vi "ULx Write (Digital Wfm 1Chan 1Samp).vi"(0 "task in":refnum<k24>, 1 "auto start":bool=TRUE, 7 "data":digitalwaveform(waveform)={"t0"=timestamp(0 s since 1904-01-01), "dt"=0.0, "Y"={"transitions"=[], "data"=[]}, "error"={"status"=FALSE, "code"=37421928, "source"=""}}, 9 "timeout":dbl=10.0 format="%_4g", 11 "error in":errorcluster) -> (4 "task out":refnum<k24>, 10 "number of samples written per channel":u32, 15 "error out":errorcluster)   [LabVIEW 2020]
doc: "Writes a digital waveform that contains a single sample to a task that contains a single digital output channel."
uses:
  C:/Users/William/Documents/LV 2020 builds/LeaktestDAQ/Source-v33/ULx_LV.dll
  ULx_LV.dll
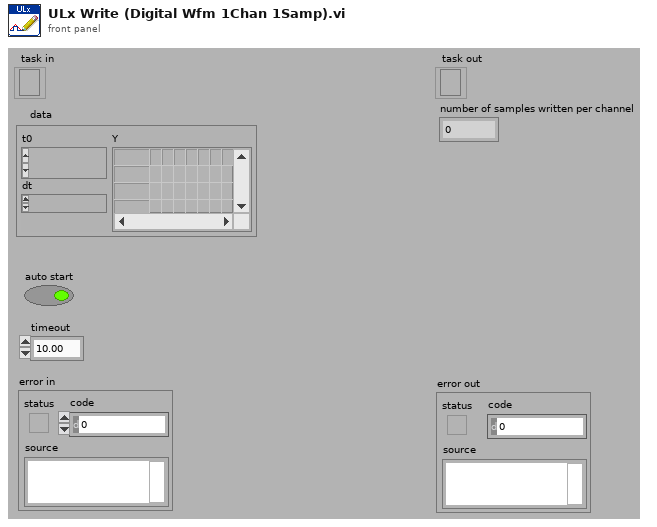
[diagram p1: front panel]
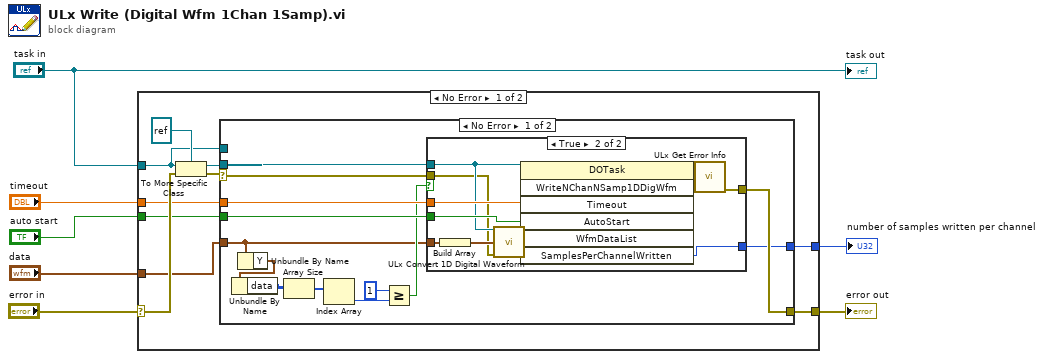
[diagram p0: block diagram]
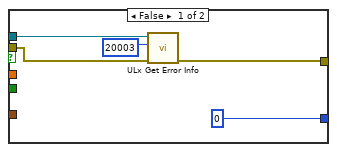
[diagram p2: hidden frame]
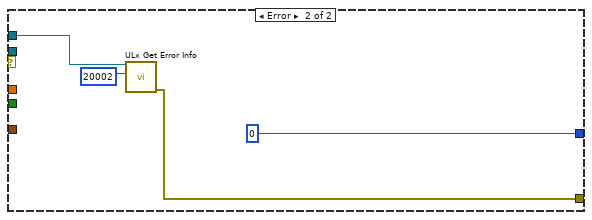
[diagram p3: hidden frame]
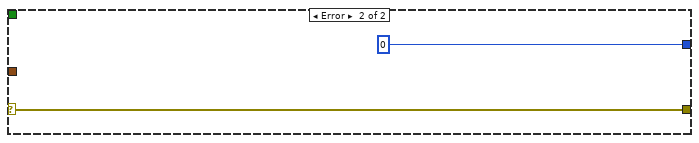
[diagram p4: hidden frame]
diagram:
  n1 = case shown="No Error" "error in" {
    selector: "error in" -> [w17 w53]
    tunnel: "task in" -> [w11 _]
    tunnel: "timeout" -> [w13 _]
    tunnel: [w12 w53] -> w5
    tunnel: "auto start" -> [w10 _]
    tunnel: [w9 0 ("SamplesPerChannelWritten")] -> w2
    tunnel: "data" -> [w8 _]
    frame No Error {
      n2 = To More Specific Class(target class=refnum<k24> refnum, reference=w11, error in=w17) -> (specific class reference=w14:refnum<k24>, error out=w15:errorcluster)
      n3 = case shown="No Error" w15 {
        selector: w15 -> [w25 _]
        tunnel: w14 -> [w26 _]
        tunnel: w13 -> [w28 _]
        tunnel: [w30 w50] -> w12
        tunnel: w11 -> [_ w49]
        tunnel: w10 -> [w27 _]
        tunnel: [w29 0 ("SamplesPerChannelWritten")] -> w9
        tunnel: w8 -> [w18 _]
        frame No Error {
          n4 = Unbundle By Name(w18) -> ("Y"=w21:digitaldata)
          n5 = Unbundle By Name(w21) -> ("data"=w24:u8[][])
          n6 = Array Size(array=w24) -> (size(s)=w23:i32[])
          n7 = Index Array(array=w23) -> (element=w20:i32)  [unwired: 1 in]
          n8 = Greater Or Equal?(x=1 ("y"), y=w20) -> (x >= y?=w22:bool)
          n9 = case shown="True" w22 {
            tunnel: [w32 w45] -> w30
            tunnel: [u32 0 ("SamplesPerChannelWritten") w43] -> w29
            tunnel: w28 -> [_ w42]
            tunnel: w27 -> [_ w41]
            tunnel: w26 -> [w34 w38]
            tunnel: w25 -> [w33 w37]
            tunnel: w18 -> [_ w40]
            frame False {
              n10 = call "ULx Get Error Info.vi"("error in"=w33, "ErrorCode"=20003, "task in"=w34) -> ("error out"=w32:errorcluster)  [unwired: 8 in]
            }
            frame True {
              n11 = Build Array(w40) -> (w39:digitalwaveform[])
              n12 = call "ULx Convert 1D Digital Waveform.vi"("task in"=w38, "data"=w39, "error in"=w37) -> ("data List"=w36:refnum<k24>)  [unwired: 11 in, 1 out]
              n13 = invoke class="DOTask" method="WriteNChanNSamp1DDigWfm"(reference=w38, "Timeout"=w42, "AutoStart"=w41, "WfmDataList"=w36) -> (reference out=w46:refnum<k24>, error out=w47:errorcluster, "WriteNChanNSamp1DDigWfm"=w44:i32, "SamplesPerChannelWritten"=w43:u32)  [unwired: 3 in, 3 out]
              n14 = call "ULx Get Error Info.vi"("error in"=w47, "ErrorCode"=w44, "task in"=w46) -> ("error out"=w45:errorcluster)  [unwired: 8 in]
            }
          }
        }
        frame Error {
          n15 = call "ULx Get Error Info.vi"("ErrorCode"=20002, "task in"=w49) -> ("error out"=w50:errorcluster)  [unwired: 9 in]
        }
      }
    }
    frame Error {
    }
  }
  "error out" <- w5
  "number of samples written per channel" <- w2
  "task out" <- "task in"
